vi "AvoidOwnGoal.vi"(0 "DefendAreaSkill in":refnum<class "DefendAreaSkill.lvclass">, 1 "Field":refnum<class "Field.lvclass">, 3 "Robot":refnum<class "Robot.lvclass">, 5 "error in (no error)":errorcluster) -> (14 "DefendAreaSkill out":refnum<class "DefendAreaSkill.lvclass">, 16 "Is shooting to our goal?":bool, 19 "error out":errorcluster)   [LabVIEW 2024, in "DefendAreaSkill.lvclass"]
uses:
  DefendAreaSkill.lvclass
  Robot_class/Robot.lvclass
  C:/Users/ROBOIME2/Documents/SSL ROBOIME/SSL_AI/Object_class/Object.lvclass
  Field_class/Field.lvclass
  Object_class/Object.lvclass/Object.ctl
  Robot_class/Robot.lvclass/Robot.ctl
  Object_class/Read x.vi
  Object_class/Read y.vi
  Robot_class/Read orientation.vi
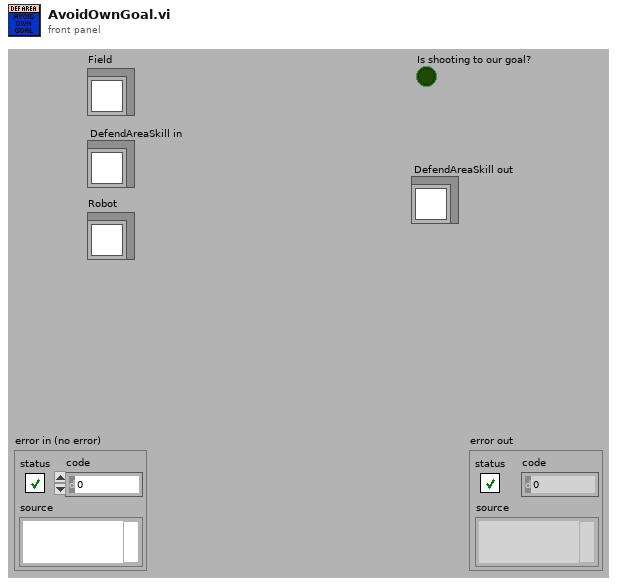
[diagram p1: front panel]
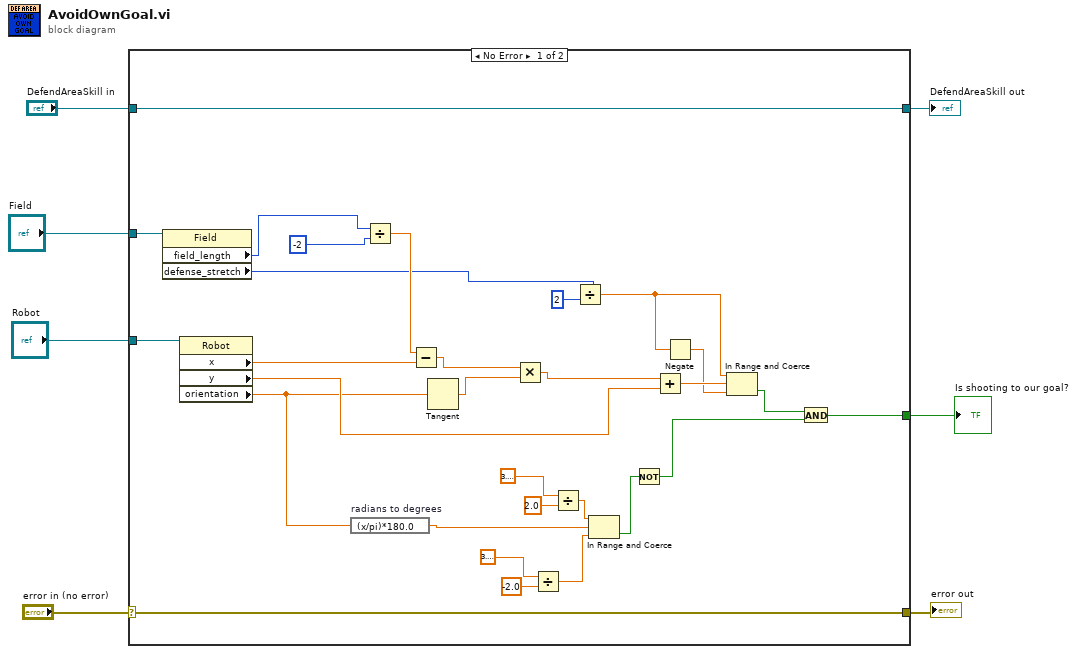
[diagram p0: block diagram]
diagram:
  n1 = case shown="No Error" "error in (no error)" {
    selector: "error in (no error)" -> [w35 w38]
    tunnel: [w35 w38] -> w6
    tunnel: [w36 w37] -> w4
    tunnel: "DefendAreaSkill in" -> [w36 w37]
    tunnel: "Robot" -> [w34 _]
    tunnel: "Field" -> [w26 _]
    tunnel: [w11 _] -> w1
    frame No Error {
      n2 = property class="Field"(reference=w26) -> ("field_length"=w25:i32, "defense_stretch"=w24:i32)  [unwired: 1 in, 2 out]
      n3 = property class="Robot"(reference=w34) -> ("x"=w33:dbl, "y"=w28:dbl, "orientation"=w19:dbl)  [unwired: 1 in, 2 out]
      n4 = expression code="(x/pi)*180.0" "radians to degrees"(w19) -> (w18:dbl)
      n5 = Divide(x=w25, y=-2) -> (x/y=w32:dbl)
      n6 = Subtract(x=w32, y=w33) -> (x-y=w31:dbl)
      n7 = Tangent(1:w19) -> (0:w30:dbl)
      n8 = Multiply(x=w31, y=w30) -> (x*y=w29:dbl)
      n9 = Divide(x=3.141592653589793, y=-2.0) -> (x/y=w13:dbl)
      n10 = Divide(x=3.141592653589793, y=2.0) -> (x/y=w12:dbl)
      n11 = Divide(x=w24, y=2) -> (x/y=w22:dbl)
      n12 = In Range and Coerce(upper limit=w12, x=w18, lower limit=w13) -> (In Range?=w8:bool)  [unwired: 1 out]
      n13 = Not(x=w8) -> (.not. x?=w9:bool)
      n14 = Add(x=w29, y=w28) -> (x+y=w27:dbl)
      n15 = Negate(x=w22) -> (-x=w21:dbl)
      n16 = In Range and Coerce(upper limit=w22, x=w27, lower limit=w21) -> (In Range?=w20:bool)  [unwired: 1 out]
      n17 = And(x=w20, y=w9) -> (x .and. y?=w11:bool)
    }
    frame Error {
    }
  }
  "error out" <- w6
  "DefendAreaSkill out" <- w4
  "Is shooting to our goal?" <- w1
